vi "UpdatePortHTMLPage.vi"(2 "Array":i32[](array[numeric]), 3 "LogPath in":path) -> (1 "LogPath out":path)   [LabVIEW 2016]
doc: "Updates HTML page with ports"
panel:
  out "concatenated string":string
  out "text":string
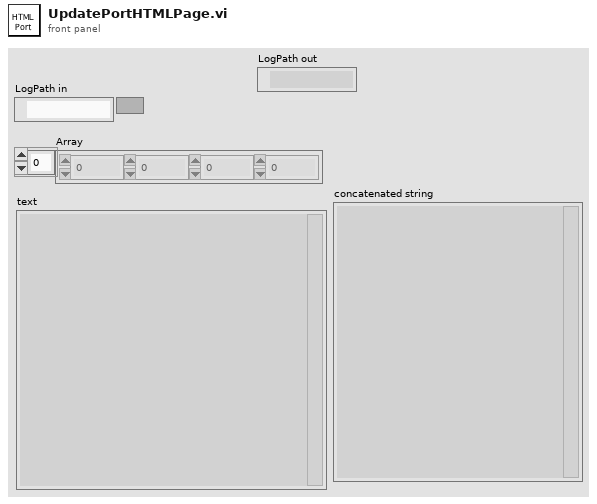
[diagram p1: front panel]
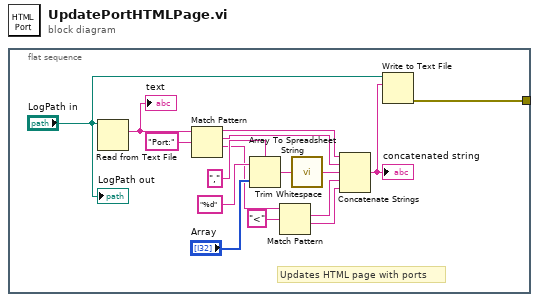
[diagram p0: block diagram]
diagram:
  n1 = flat-sequence {
    tunnel: [w1] -> _
    frame #0 {
      # "Updates HTML page with ports"
      n2 = Read from Text File(file (use dialog)="LogPath in") -> (text=w9:string)  [unwired: 3 in, 3 out]
      "text" <- w9
      n3 = Match Pattern(string=w9, regular expression="Port:") -> (before substring=w14:string, match substring=w5:string, after substring=w10:string)  [unwired: 1 in, 1 out]
      n4 = Array To Spreadsheet String(delimiter (Tab)=",", array="Array", 3:"%d" ("format string")) -> (spreadsheet string=w15:string)
      n5 = Match Pattern(string=w10, regular expression="<") -> (match substring=w4:string, after substring=w7:string)  [unwired: 1 in, 2 out]
      n6 = call "Trim Whitespace.vi"("string"=w15) -> ("trimmed string"=w3:string)  [unwired: 1 in]
      n7 = Concatenate Strings(w14, w5, w3, w4, w7) -> (w16:string)
      "concatenated string" <- w16
      n8 = Write to Text File(file (use dialog)="LogPath in", text=w16) -> (error out=w1:errorcluster)  [unwired: 2 in, 2 out]
      "LogPath out" <- "LogPath in"
    }
  }
